vi "DHE_SetObsParams.vi"(10 "DHE_OBS":T1={"observer"="", "obstype"="", "exptime"=0.0, "coadds"=1, "fowler"=1, "nimages"=0, "display"=TRUE, "autowrite"=TRUE, "frames to write"={"subs"=TRUE, "reset"=FALSE, "exposed"=FALSE}, "frames to display"={"subs"=TRUE, "reset"=FALSE, "exposed"=FALSE}, "sur"=0} {"exptime" format="%.2f"}) -> ()   [LabVIEW 2016]
uses:
  private/vis/DHE_Obs.ctl
  Common/public/vis/CMN_FVAR_action.ctl
  DBSHAND/private/vis/DatabaseHand_Element_Set(string).vi
  DBSHAND/private/vis/DatabaseHand_Element_Set(double).vi
  DBSHAND/private/vis/DatabaseHand_Element_Set(I32).vi
  DBSHAND/private/vis/DatabaseHand_Element_Set(bool).vi
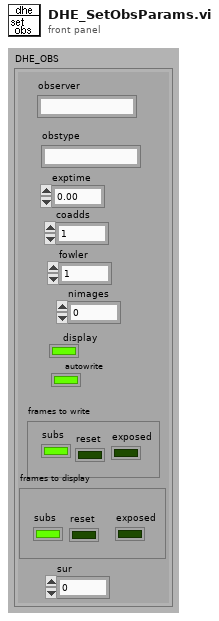
[diagram p1: front panel]
types:
  T1 = typedef "DHE_Obs.ctl" = cluster{"observer":string, "obstype":string, "exptime":dbl, "coadds":i32, "fowler":i32, "nimages":i32, "display":bool, "autowrite":bool, "frames to write":cluster{"subs":bool, "reset":bool, "exposed":bool}, "frames to display":cluster{"subs":bool, "reset":bool, "exposed":bool}, "sur":i32}
  T2 = typedef "CMN_FVAR_action.ctl" = enum16{"read", "write"}
  T3 = typedef "DatabaseHand_RefNum.ctl" = refnum<vi>
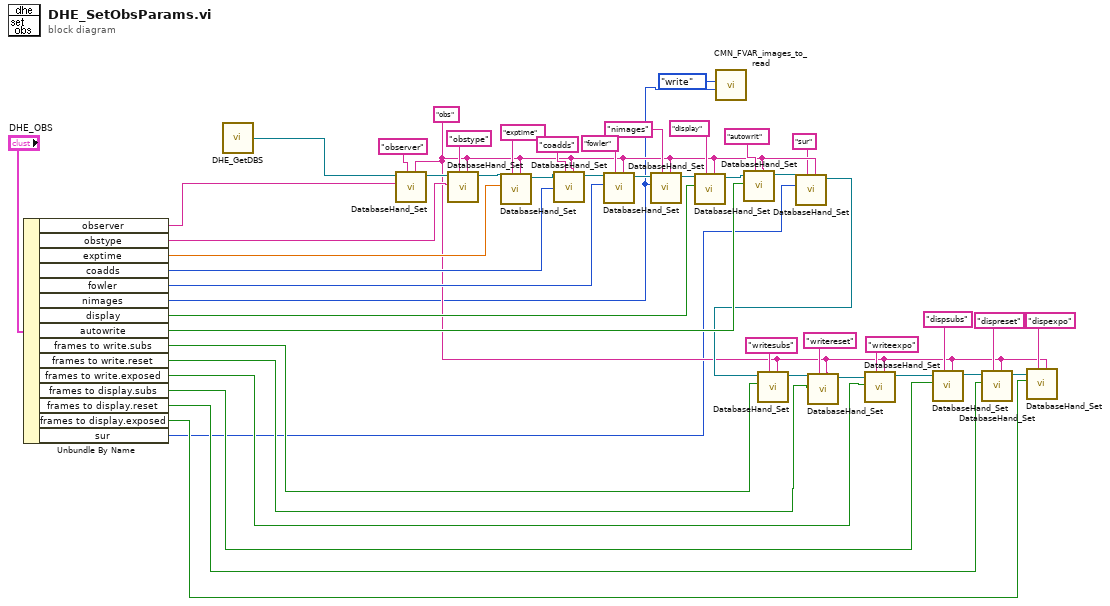
[diagram p0: block diagram]
diagram:
  w6 = "obs" ("group")
  n1 = Unbundle By Name("DHE_OBS") -> ("observer"=w47:string, "obstype"=w42:string, "exptime"=w40:dbl, "coadds"=w38:i32, "fowler"=w18:i32, "nimages"=w2:i32, "display"=w20:bool, "autowrite"=w36:bool, "frames to write.subs"=w33:bool, "frames to write.reset"=w31:bool, "frames to write.exposed"=w29:bool, "frames to display.subs"=w11:bool, "frames to display.reset"=w10:bool, "frames to display.exposed"=w9:bool, "sur"=w4:i32)
  n2 = call "DHE_GetDBS.vi"() -> ("DHE_DBSRef"=w3:T3)  [unwired: 9 out]
  n3 = call-poly "DatabaseHand_Set.vi"("group"=w6, "name"="observer", "value"=w47, "Database RefNum in"=w3) -> ("Database RefNum out"=w46:T3)  [unwired: 4 in, 3 out]
  n4 = call-poly "DatabaseHand_Set.vi"("group"=w6, "name"="obstype", "value"=w42, "Database RefNum in"=w46) -> ("Database RefNum out"=w45:T3)  [unwired: 4 in, 3 out]
  n5 = call-poly "DatabaseHand_Set.vi"("group"=w6, "name"="exptime", "value"=w40, "Database RefNum in"=w45) -> ("Database RefNum out"=w44:T3)  [unwired: 4 in, 3 out]
  n6 = call-poly "DatabaseHand_Set.vi"("group"=w6, "name"="coadds", "value"=w38, "Database RefNum in"=w44) -> ("Database RefNum out"=w43:T3)  [unwired: 4 in, 3 out]
  n7 = call-poly "DatabaseHand_Set.vi"("group"=w6, "name"="fowler", "value"=w18, "Database RefNum in"=w43) -> ("Database RefNum out"=w25:T3)  [unwired: 4 in, 3 out]
  n8 = call-poly "DatabaseHand_Set.vi"("group"=w6, "name"="nimages", "value"=w2, "Database RefNum in"=w25) -> ("Database RefNum out"=w24:T3)  [unwired: 4 in, 3 out]
  n9 = call-poly "DatabaseHand_Set.vi"("group"=w6, "name"="display", "value"=w20, "Database RefNum in"=w24) -> ("Database RefNum out"=w23:T3)  [unwired: 4 in, 3 out]
  n10 = call "CMN_FVAR_images_to_read.vi"("value in"=w2, "action"=CMN_FVAR_action."write") -> ()  [unwired: 9 out]
  n11 = call-poly "DatabaseHand_Set.vi"("group"=w6, "name"="autowrit", "value"=w36, "Database RefNum in"=w23) -> ("Database RefNum out"=w8:T3)  [unwired: 4 in, 3 out]
  n12 = call-poly "DatabaseHand_Set.vi"("group"=w6, "name"="sur", "value"=w4, "Database RefNum in"=w8) -> ("Database RefNum out"=w7:T3)  [unwired: 4 in, 3 out]
  n13 = call-poly "DatabaseHand_Set.vi"("group"=w6, "name"="writesubs", "value"=w33, "Database RefNum in"=w7) -> ("Database RefNum out"=w28:T3)  [unwired: 4 in, 3 out]
  n14 = call-poly "DatabaseHand_Set.vi"("group"=w6, "name"="writereset", "value"=w31, "Database RefNum in"=w28) -> ("Database RefNum out"=w27:T3)  [unwired: 4 in, 3 out]
  n15 = call-poly "DatabaseHand_Set.vi"("group"=w6, "name"="writeexpo", "value"=w29, "Database RefNum in"=w27) -> ("Database RefNum out"=w14:T3)  [unwired: 4 in, 3 out]
  n16 = call-poly "DatabaseHand_Set.vi"("group"=w6, "name"="dispsubs", "value"=w11, "Database RefNum in"=w14) -> ("Database RefNum out"=w13:T3)  [unwired: 4 in, 3 out]
  n17 = call-poly "DatabaseHand_Set.vi"("group"=w6, "name"="dispreset", "value"=w10, "Database RefNum in"=w13) -> ("Database RefNum out"=w12:T3)  [unwired: 4 in, 3 out]
  n18 = call-poly "DatabaseHand_Set.vi"("group"=w6, "name"="dispexpo", "value"=w9, "Database RefNum in"=w12) -> ()  [unwired: 4 in, 4 out]
